vi "subApplyFrequencyCorrection.vi"(0 "input signal":cdb[](array[numeric]) format="%#_6p", 5 "phase shift (rad/point)":dbl format="%#_6p", 11 "error in (no error)":errorcluster) -> (4 "output signal":cdb[](array[numeric]) format="%#_6p", 15 "error out":errorcluster)   [LabVIEW 2011]
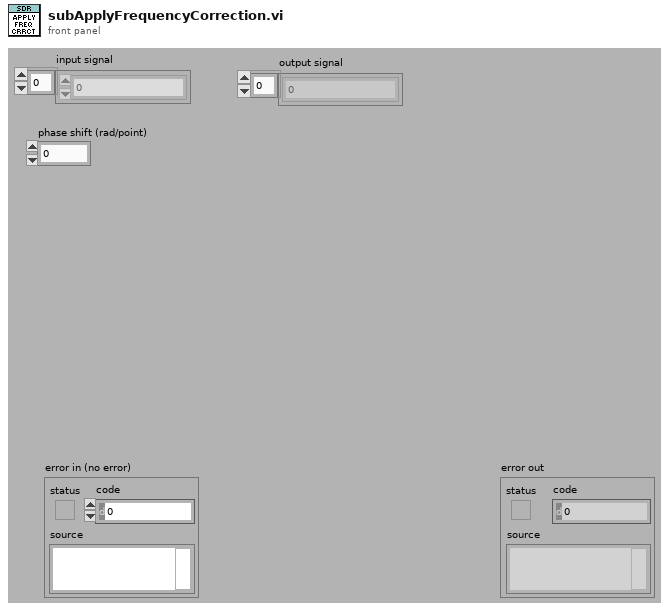
[diagram p1: front panel]
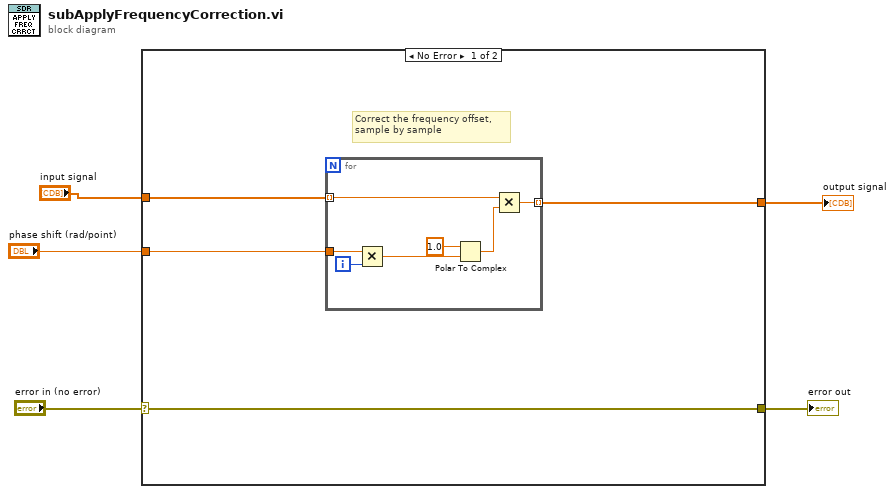
[diagram p0: block diagram]
diagram:
  n1 = case shown="No Error" "error in (no error)" {
    selector: "error in (no error)" -> [w9 w18]
    tunnel: [w9 w18] -> w4
    tunnel: "input signal" -> [w8 w17]
    tunnel: "phase shift (rad/point)" -> [w7 _]
    tunnel: [w6 w17] -> w1
    frame No Error {
      # "Correct the frequency offset, \nsample by sample"
      n2 = for {
        tunnel: w8 -> [w13] mode=indexing
        tunnel: w7 -> [w15]
        tunnel: [w11] -> w6 mode=indexing
        i -> [w16]
        n3 = Multiply(x=w15, y=w16) -> (x*y=w10:dbl)
        n4 = Polar To Complex(1:w10, 2:1.0 ("r")) -> (0:w12:cdb)
        n5 = Multiply(x=w13, y=w12) -> (x*y=w11:cdb)
      }
    }
    frame Error {
    }
  }
  "error out" <- w4
  "output signal" <- w1
